vi "Read description.vi"(8 "error in (no error)":errorcluster, 11 "ExampleTask_MsgUserEventStopNotifier In":refnum<class "ExampleTask_MsgUserEventStopNotifier.lvclass">) -> (0 "error out":errorcluster, 2 "description":string, 3 "ExampleTask_MsgUserEventStopNotifier Out":refnum<class "ExampleTask_MsgUserEventStopNotifier.lvclass">)   [LabVIEW 2023, in "ExampleTask_MsgUserEventStopNotifier.lvclass"]
uses:
  ExampleTask_MsgUserEventStopNotifier.lvclass
  ExampleTask_MsgUserEventStopNotifier.lvclass/ExampleTask_MsgUserEventStopNotifier.ctl
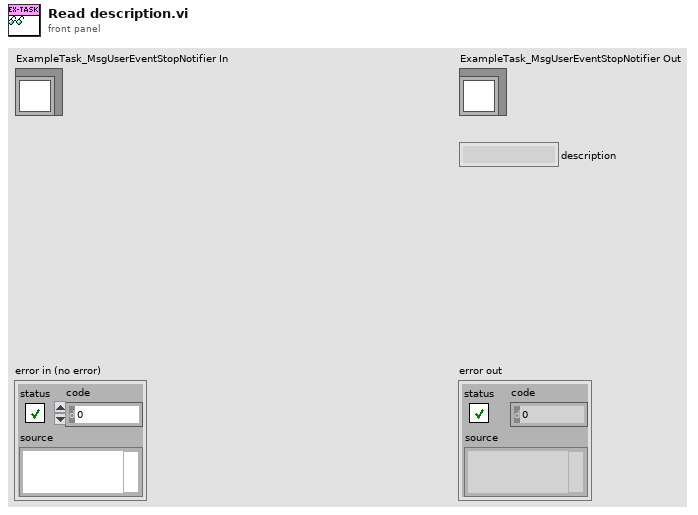
[diagram p1: front panel]
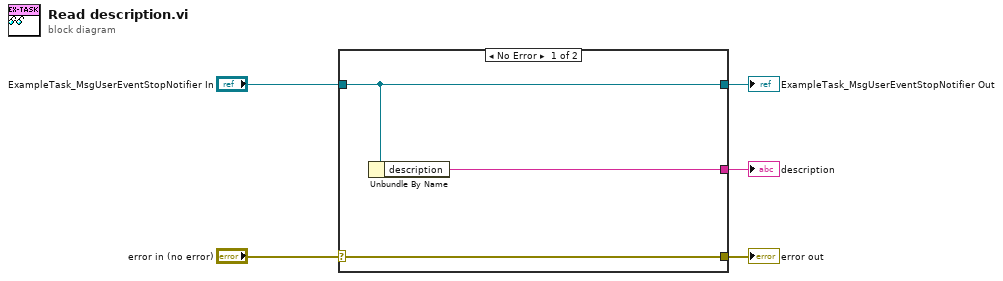
[diagram p0: block diagram]
diagram:
  n1 = case shown="No Error" "error in (no error)" {
    selector: "error in (no error)" -> [w8 w9]
    tunnel: [w8 w9] -> w4
    tunnel: [w7 w10] -> w2
    tunnel: "ExampleTask_MsgUserEventStopNotifier In" -> [w7 w10]
    tunnel: [w6 _] -> w1
    frame No Error {
      n2 = Unbundle By Name(w7) -> ("description"=w6:string)
    }
    frame Error {
    }
  }
  "error out" <- w4
  "ExampleTask_MsgUserEventStopNotifier Out" <- w2
  "description" <- w1
